vi "Public Key File Authentication.vi"(4 "Key Files":cluster{"Private":path, "Public":path}={"Private"=path "", "Public"=path ""}, 5 "Username":string, 6 "Passphrase":string, 7 "Address":string, 8 "Error In":errorcluster) -> (0 "Error Out":errorcluster)   [LabVIEW 2018, in "Tests.lvlib" / "Session.lvlib"]
uses:
  Session.lvlib
  Support/SSH Key Types.ctl
  Support/Secret Types.ctl
  <vilib>/Utility/file.llb/Is Path and Not Empty.vi
  <vilib>/Utility/sysdir.llb/Get System Directory.vi
  <vilib>/addons/_JKI Toolkits/Caraya/classes/Test/Test.lvclass
  src/Toolkit/API/SSH/SSH.lvclass
  src/Toolkit/API/Session/Session.lvclass
  <vilib>/addons/_JKI Toolkits/Caraya/classes/Assert/Assert.lvclass
  Tests.lvlib
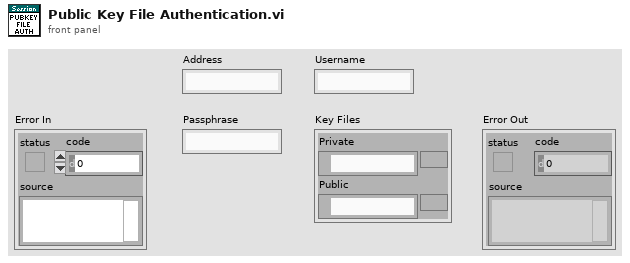
[diagram p1: front panel]
types:
  T1 = typedef "Tests.lvlib/SSH Key Types.ctl" = enum16{"Private", "Public"}
  T2 = typedef "Tests.lvlib/Secret Types.ctl" = enum16{"Passphrase", "Password"}
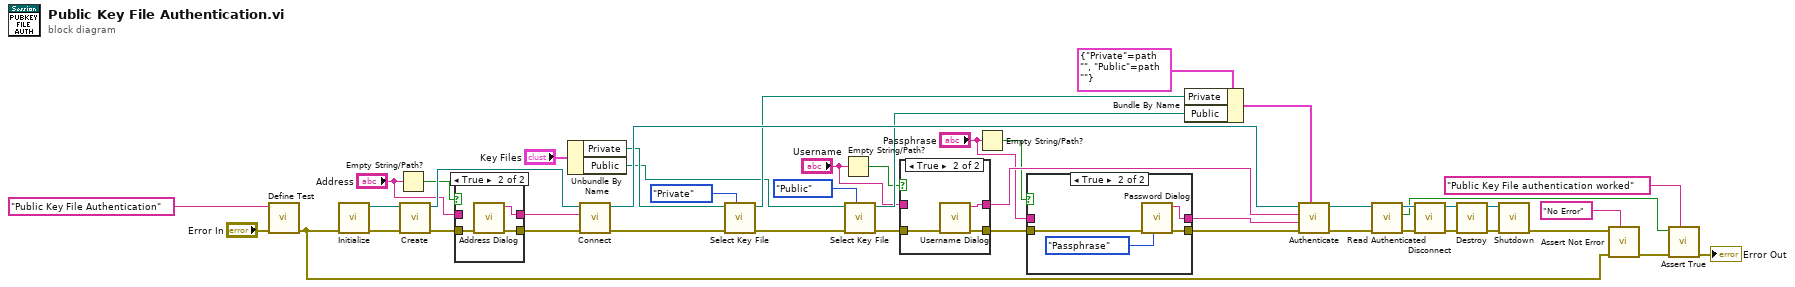
[diagram p0: block diagram]
diagram:
  n1 = call <vilib>:"Define Test.vi"("error in (no error)"="Error In", "Label (VI Title)"="Public Key File Authentication") -> ("error out"=w38:errorcluster)  [unwired: 9 in]
  n2 = call "Initialize.vi"("Error In"=w38) -> ("Error Out"=w44:errorcluster, "SSH"=w43:refnum<class "SSH.lvclass">)  [unwired: 9 in]
  n3 = Empty String/Path?(string/path="Address") -> (empty?=w17:bool)
  n4 = call "Create.vi"("Error In"=w44, "SSH"=w43) -> ("Error Out"=w16:errorcluster, "Sesssion"=w36:refnum<class "Session.lvclass">)  [unwired: 8 in]
  n5 = case shown="True" w17 {
    tunnel: w16 -> [w47 w51]
    tunnel: [w47 w50] -> w15
    tunnel: [w48 w49] -> w14
    tunnel: "Address" -> [w48 _]
    frame False {
    }
    frame True {
      n6 = call "Address Dialog.vi"("Error In"=w51) -> ("Error Out"=w50:errorcluster, "Address Out"=w49:string)  [unwired: 9 in]
    }
  }
  n7 = Unbundle By Name("Key Files") -> ("Private"=w2:path, "Public"=w1:path)
  n8 = call "Connect.vi"("Error In"=w15, "Address"=w14, "Session In"=w36) -> ("Error Out"=w24:errorcluster, "Sesssion Out"=w33:refnum<class "Session.lvclass">)  [unwired: 7 in]
  n9 = call "Select Key File.vi"("Key Type"=SSH_Key_Types."Private", "Error In"=w24, "Key File In"=w2) -> ("Error Out"=w20:errorcluster, "Key File Out"=w21:path)  [unwired: 7 in]
  n10 = Empty String/Path?(string/path="Username") -> (empty?=w12:bool)
  n11 = call "Select Key File.vi"("Key Type"=SSH_Key_Types."Public", "Error In"=w20, "Key File In"=w1) -> ("Error Out"=w9:errorcluster, "Key File Out"=w19:path)  [unwired: 7 in]
  n12 = case shown="True" w12 {
    tunnel: [w53 w56] -> w11
    tunnel: "Username" -> [w53 _]
    tunnel: w9 -> [w52 w55]
    tunnel: [w52 w54] -> w7
    frame False {
    }
    frame True {
      n13 = call "Username Dialog.vi"("Error In"=w55) -> ("Error Out"=w54:errorcluster, "Username Out"=w56:string)  [unwired: 9 in]
    }
  }
  n14 = Empty String/Path?(string/path="Passphrase") -> (empty?=w8:bool)
  n15 = case shown="True" w8 {
    tunnel: w7 -> [w57 w62]
    tunnel: "Passphrase" -> [w58 _]
    tunnel: [w58 w61] -> w5
    tunnel: [w57 w60] -> w4
    frame False {
    }
    frame True {
      n16 = call "Password Dialog.vi"("Secret Type"=Secret_Types."Passphrase", "Error In"=w62) -> ("Error Out"=w60:errorcluster, "Password Out"=w61:string)  [unwired: 8 in]
    }
  }
  n17 = Bundle By Name(cluster=cluster{"Private":path, "Public":path} {"Private"=path "", "Public"=path ""} ("Keys"), "Private"=w21, "Public"=w19) -> (w22:cluster{"Private":path, "Public":path})
  n18 = call-poly "Authenticate.vi"("Keys"=w22, "Error In"=w4, "Passphrase"=w5, "Username"=w11, "Session In"=w33) -> ("Error Out"=w31:errorcluster, "Sesssion Out"=w32:refnum<class "Session.lvclass">)  [unwired: 5 in]
  n19 = call "Read Authenticated.vi"("Error In"=w31, "Session In"=w32) -> ("Error Out"=w30:errorcluster, "Authenticated"=w27:bool, "Sesssion Out"=w29:refnum<class "Session.lvclass">)  [unwired: 7 in]
  n20 = call "Disconnect.vi"("Error In"=w30, "Session In"=w29) -> ("Error Out"=w34:errorcluster, "Sesssion Out"=w35:refnum<class "Session.lvclass">)  [unwired: 8 in]
  n21 = call "Destroy.vi"("Error In"=w34, "Session"=w35) -> ("Error Out"=w41:errorcluster, "SSH"=w42:refnum<class "SSH.lvclass">)  [unwired: 8 in]
  n22 = call "Shutdown.vi"("Error In"=w41, "SSH"=w42) -> ("Error Out"=w40:errorcluster)  [unwired: 9 in]
  n23 = call <vilib>:"Assert Not Error.vi"("Label"="No Error", "error in (no error)"=w38, "Not Error?"=w40) -> ("error out"=w37:errorcluster)  [unwired: 8 in]
  n24 = call <vilib>:"Assert True.vi"("Label"="Public Key File authentication worked", "error in (no error)"=w37, "True?"=w27) -> ("error out"=→"Error Out":errorcluster)  [unwired: 8 in]
